vi "angle_between_vectors.vi"(1 "vector 2":cluster{"X":dbl, "Y":dbl}, 2 "vector 1":cluster{"X":dbl, "Y":dbl}) -> (0 "arccos(x)":dbl)   [LabVIEW 2019]
uses:
  <vilib>/Analysis/baseanly.llb/Real Dot Product.vi
  euclidean_distance.vi
  <vilib>/Analysis/NI_AALBase.lvlib
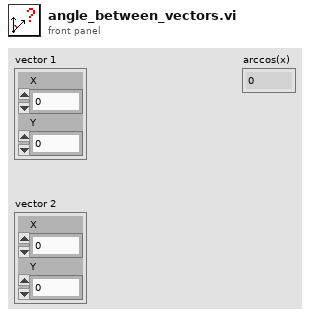
[diagram p1: front panel]
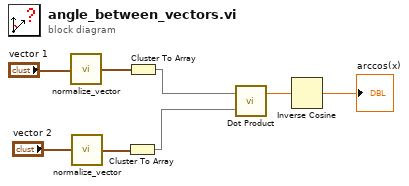
[diagram p0: block diagram]
diagram:
  n1 = call "normalize_vector.vi"("vector"="vector 1") -> ("normalized vector"=w6:cluster{"X":dbl, "Y":dbl})
  n2 = call "normalize_vector.vi"("vector"="vector 2") -> ("normalized vector"=w4:cluster{"X":dbl, "Y":dbl})
  n3 = Cluster To Array(cluster=w4) -> (array=w3:dbl[])
  n4 = Cluster To Array(cluster=w6) -> (array=w5:dbl[])
  n5 = call-poly <vilib>:"Dot Product.vi"("Y Vector"=w3, "X Vector"=w5) -> ("X * Y"=w2:dbl)  [unwired: 1 out]
  n6 = Inverse Cosine(1:w2) -> (0:→"arccos(x)":dbl)
